vi "Phasor Abort Parallel Computation.vi"() -> ()   [LabVIEW 2021, in "Phasor.lvlib"]
uses:
  Phasor.lvlib
panel:
  out "Abort Parallel Computation":bool
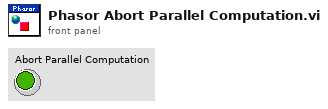
[diagram p1: front panel]
diagram:
